vi "InterpCPUUsage.vi"(7 "Idle":dbl, 8 "Time Critical":dbl, 9 "High":dbl, 10 "Normal":dbl, 11 "Low":dbl) -> (0 "Low Priority":dbl, 1 "Normal Priority":dbl, 2 "High Priority":dbl, 3 "Time Critical":dbl)   [LabVIEW 2010, in "kevLib2010.lvlib"]
uses:
  kevLib2010.lvlib
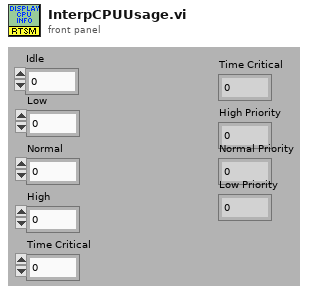
[diagram p1: front panel]
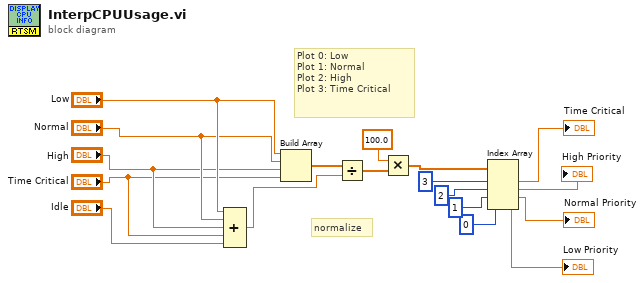
[diagram p0: block diagram]
diagram:
  # "normalize"
  # "Plot 0: Low\nPlot 1: Normal\nPlot 2: High\nPlot 3: Time Critical"
  n1 = Compound Arithmetic op=ADD("Low", "Normal", "High", "Time Critical", "Idle") -> (w1:dbl)
  n2 = Build Array("Low", "Normal", "High", "Time Critical") -> (w18:dbl[])
  n3 = Divide(x=w18, y=w1) -> (x/y=w17:dbl[])
  n4 = Multiply(x=100.0, y=w17) -> (x*y=w15:dbl[])
  n5 = Index Array(array=w15, index #1=3 ("index"), index #2=2 ("index"), index #3=1 ("index"), index #4=0 ("index")) -> (element #1=→"Time Critical":dbl, element #2=→"High Priority":dbl, element #3=→"Normal Priority":dbl, element #4=→"Low Priority":dbl)
